vi "Read Write scaling configuration.vi"(4 "error in":errorcluster, 5 "Input":T1(array[cluster]), 6 "Read/Write":u16(ring) items=["READ", "WRITE"]) -> (0 "error out":errorcluster, 1 "Output":T1(array[cluster]), 2 "Numeric":i32)   [LabVIEW 2015]
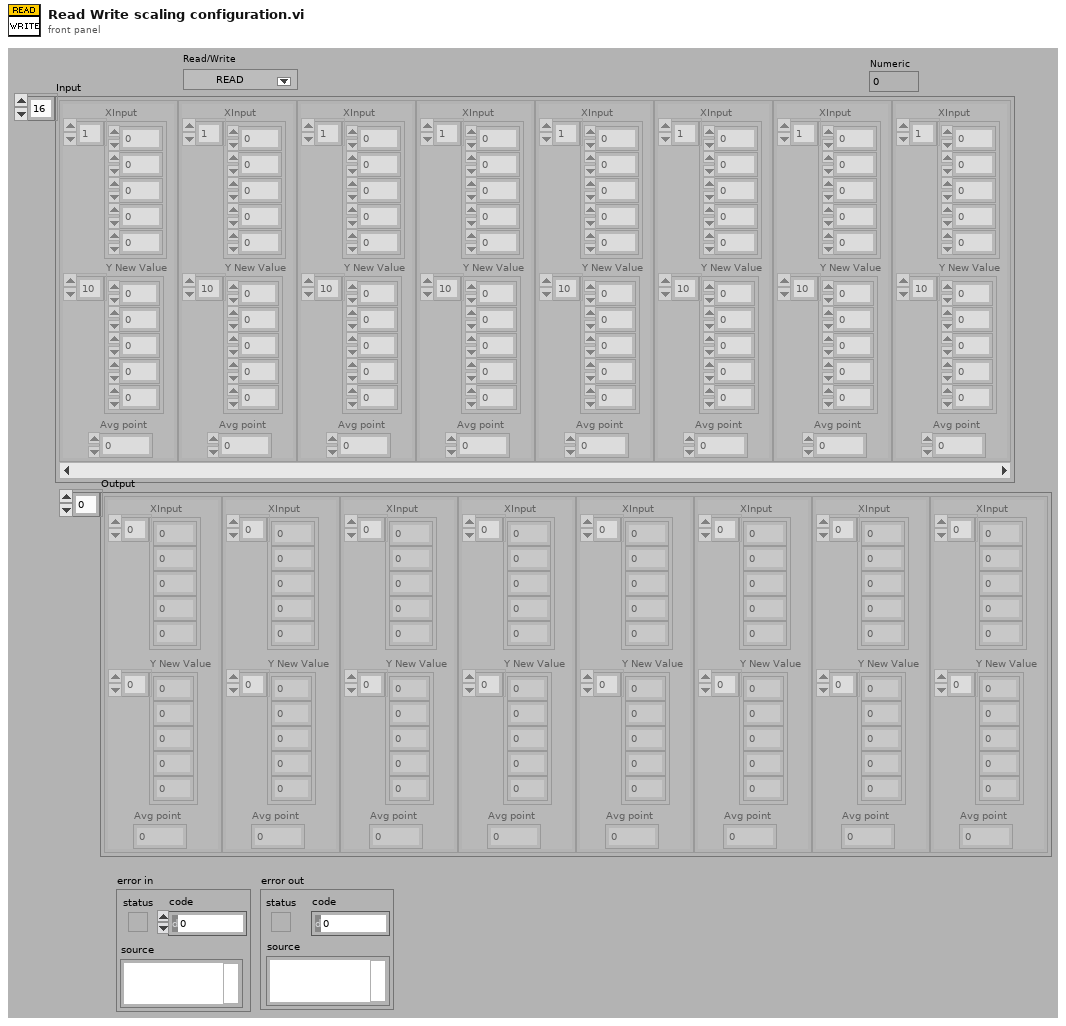
[diagram p1: front panel]
types:
  T1 = cluster{"XInput":dbl[], "Y New Value":dbl[], "Avg point":i16}[]
  T2 = enum16{"open", "replace", "create", "open or create", "replace or create", "replace or create with confirmation"}
  T3 = enum16{"read/write", "read-only", "write-only", "write-only (truncate)"}
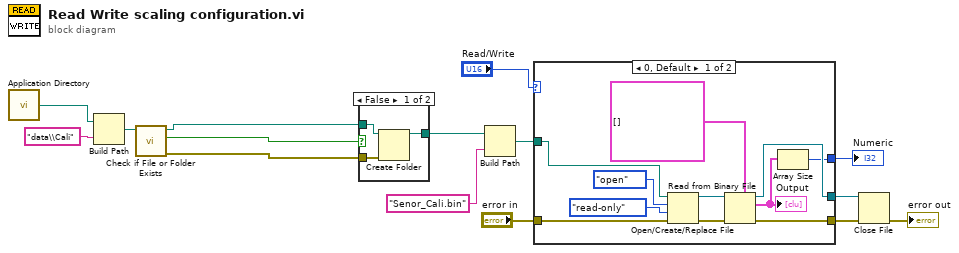
[diagram p0: block diagram]
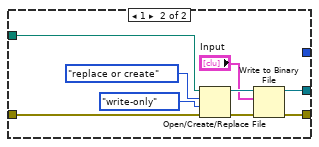
[diagram p3: hidden frame]
diagram:
  n1 = call <vilib>:"Application Directory.vi"() -> ("Application Directory"=w9:path)
  n2 = Build Path(base path=w9, name or relative path="data\\Cali") -> (appended path=w5:path)
  n3 = call <vilib>:"Check if File or Folder Exists.vi"("path"=w5) -> ("error out"=w3:errorcluster, "file or folder exists?"=w4:bool, "dup path"=w2:path)  [unwired: 8 in]
  n4 = case shown="False" w4 {
    tunnel: w3 -> [w18 _]
    tunnel: w2 -> [w17 w19]
    tunnel: [w16 w19] -> w1
    frame False {
      n5 = Create Folder(path (use dialog)=w17, error in=w18) -> (created path=w16:path)  [unwired: 1 in, 2 out]
    }
    frame True {
    }
  }
  n6 = Build Path(base path=w1, name or relative path="Senor_Cali.bin") -> (appended path=w6:path)
  n7 = case shown="0, Default" "Read/Write" {
    tunnel: [w28 w37] -> w14
    tunnel: [w27 w36] -> w13
    tunnel: w6 -> [w26 w39]
    tunnel: "error in" -> [w25 w38]
    tunnel: [w23 _] -> w10
    frame 0, Default {
      n8 = Open/Create/Replace File(file path (use dialog)=w26, error in=w25, operation (0:open)=T2."open", access (0:read/write)=T3."read-only" ("open mode (0)")) -> (refnum out=w30:refnum<file>, error out=w29:errorcluster)  [unwired: 2 in, 1 out]
      n9 = Read from Binary File(5:cluster{"X":dbl[], "Y":dbl[], "Avg point":i16}[] [] ("Output 2"), 8:w29, 11:w30) -> (0:w27:errorcluster, 2:w22:cluster{"X":dbl[], "Y":dbl[], "Avg point":i16}[], 3:w28:refnum<file>)  [unwired: 4 out]
      "Output" <- w22
      n10 = Array Size(array=w22) -> (size(s)=w23:i32)
    }
    frame 1 {
      n11 = Open/Create/Replace File(file path (use dialog)=w39, error in=w38, operation (0:open)=T2."replace or create", access (0:read/write)=enum16{"read/write", "read-only", "write-only"}."write-only") -> (refnum out=w35:refnum<file>, error out=w34:errorcluster)  [unwired: 2 in, 1 out]
      n12 = Write to Binary File(file (use dialog)=w35, data="Input", error in=w34) -> (refnum out=w37:refnum<file>, error out=w36:errorcluster)  [unwired: 4 out]
    }
  }
  "Numeric" <- w10
  n13 = Close File(refnum=w14, error in=w13) -> (error out=→"error out":errorcluster)  [unwired: 1 out]
